vi "Set Name.vi"(8 "error in (no error)":errorcluster, 10 "name":string, 11 "reference Class in":refnum<class "Reference Class.lvclass">) -> (0 "error out":errorcluster, 3 "reference Class out":refnum<class "Reference Class.lvclass">)   [LabVIEW 2023, in "Reference Class.lvclass"]
doc: "Set \"name.\""
uses:
  Reference Class.lvclass
  Reference Class.lvclass/Reference Class.ctl
  SimpleClass/Simple Class.lvclass
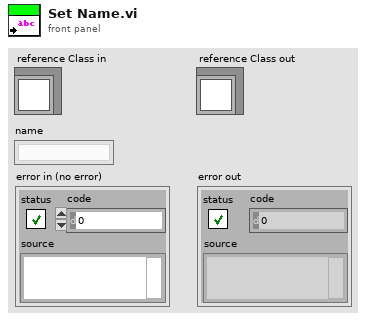
[diagram p1: front panel]
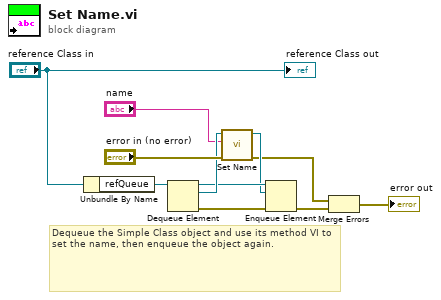
[diagram p0: block diagram]
diagram:
  # "Dequeue the Simple Class object and use its method VI to set the name, then enqueue the object again."
  n1 = Unbundle By Name("reference Class in") -> ("refQueue"=w9:refnum<queue>)
  n2 = Dequeue Element(queue=w9) -> (queue out=w7:refnum<queue>, element=w8:refnum<class "Simple Class.lvclass">, error out=w6:errorcluster)  [unwired: 2 in, 1 out]
  n3 = call "Set Name.vi"("error in (no error)"="error in (no error)", "name"="name", "simple Class in"=w8) -> ("error out"=w2:errorcluster, "simple Class out"=w5:refnum<class "Simple Class.lvclass">)  [unwired: 7 in]
  n4 = Enqueue Element(queue=w7, element=w5, error in (no error)=w6) -> (error out=w1:errorcluster)  [unwired: 1 in, 2 out]
  n5 = Merge Errors(w2, w1) -> (→"error out":errorcluster)
  "reference Class out" <- "reference Class in"
